vi "Set Next Button Visibility.vi"(8 "error in (no error)":errorcluster, 10 "Next Button Visibility":bool, 11 "Next Button Visibility Msg in":refnum<class "Next Button Visibility Msg.lvclass">) -> (0 "error out":errorcluster, 3 "Next Button Visibility Msg out":refnum<class "Next Button Visibility Msg.lvclass">)   [LabVIEW 2013, in "Project Model.lvlib" / "Next Button Visibility Msg.lvclass"]
uses:
  Next Button Visibility Msg.lvclass
  Next Button Visibility Msg.lvclass/Next Button Visibility Msg.ctl
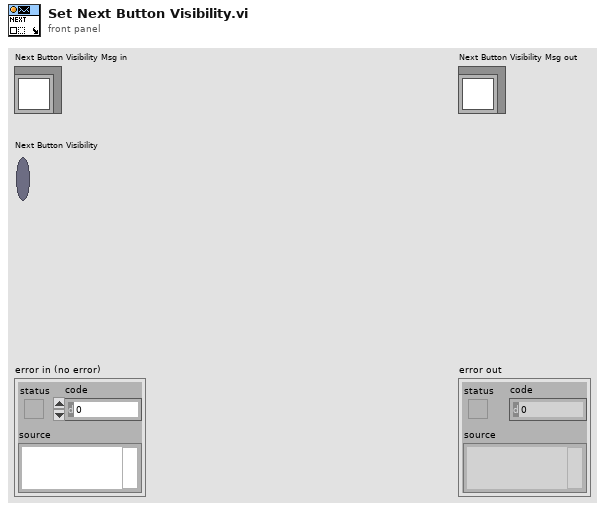
[diagram p1: front panel]
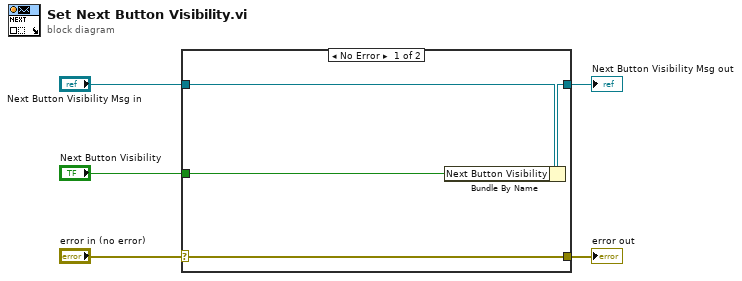
[diagram p0: block diagram]
diagram:
  n1 = case shown="No Error" "error in (no error)" {
    selector: "error in (no error)" -> [w9 w10]
    tunnel: [w9 w10] -> w4
    tunnel: [w7 w11] -> w2
    tunnel: "Next Button Visibility Msg in" -> [w8 w11]
    tunnel: "Next Button Visibility" -> [w6 _]
    frame No Error {
      n2 = Bundle By Name(cluster=w8, "Next Button Visibility"=w6) -> (w7:refnum<class "Next Button Visibility Msg.lvclass">)
    }
    frame Error {
    }
  }
  "error out" <- w4
  "Next Button Visibility Msg out" <- w2
